vi "Calculate Legend String Origin Point.vi"(8 "error in (no error)":errorcluster caption="错误输入（无错误）", 9 "origin":cluster{"x":i16, "y":i16} caption="Origin", 10 "Legend Info":T1={"Name"="", "Percent"=0.0, "TxtColor"=0, "Hor Space"=0, "Ver Space"=5, "Color Segement"=[16448250, 0, 16736786, 1198079]}, 11 "Gradient PieChart 输入":refnum<class "Gradient PieChart.lvclass"> caption="DNL_LabVIEW Object in") -> (0 "error out":errorcluster caption="错误输出", 1 "Next Origin":cluster{"x":i16, "y":i16} caption="Next Orgin", 3 "Gradient PieChart 输出":refnum<class "Gradient PieChart.lvclass"> caption="DNL_LabVIEW Object out")   [LabVIEW 2012, in "Picture Box Tools.lvlib" / "Gradient PieChart.lvclass"]
uses:
  Gradient PieChart.lvclass
  Legend Info.ctl
  Picture Box Tools.lvlib
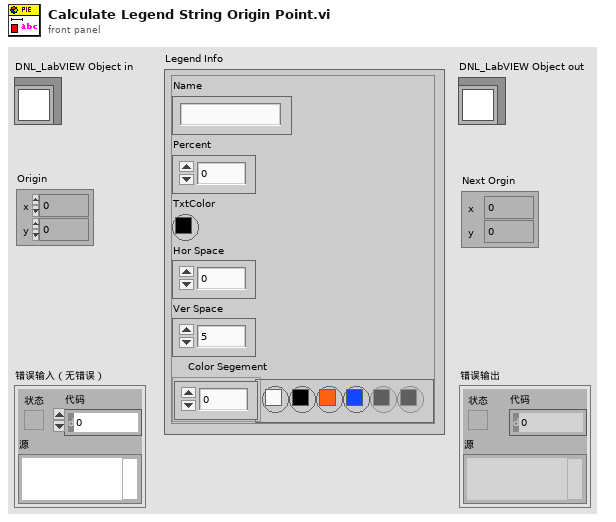
[diagram p1: front panel]
types:
  T1 = typedef "Picture Box Tools.lvlib/Gradient PieChart.lvclass/Legend Info.ctl" = cluster{"Name":string, "Percent":dbl, "TxtColor":u32, "Hor Space":i16, "Ver Space":i16, "Color Segement":u32[]}
  T2 = cluster{"left":i16, "top":i16, "right":i16, "bottom":i16}
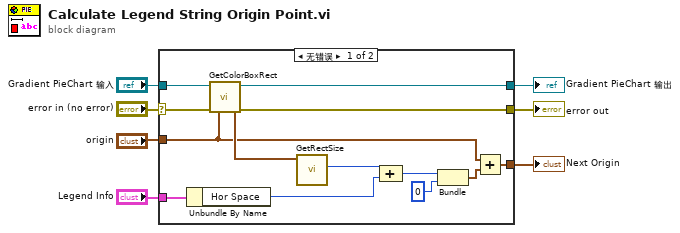
[diagram p0: block diagram]
diagram:
  n1 = case shown="无错误" "error in (no error)" {
    selector: "error in (no error)" -> [w17 w22]
    tunnel: [w16 w22] -> w6
    tunnel: [w18 w21] -> w4
    tunnel: "Gradient PieChart 输入" -> [w19 w21]
    tunnel: "Legend Info" -> [w20 _]
    tunnel: "origin" -> [w11 _]
    tunnel: [w10 _] -> w1
    frame No Error {
      n2 = Unbundle By Name(w20) -> ("Hor Space"=w14:i16)
      n3 = call "GetColorBoxRect.vi"("error in (no error)"=w17, "origin"=w11, "Gradient PieChart 输入"=w19) -> ("error out"=w16:errorcluster, "ColorBoxRect"=w15:T2, "Gradient PieChart 输出"=w18:refnum<class "Gradient PieChart.lvclass">)  [unwired: 6 in]
      n4 = call "GetRectSize.vi"("rect"=w15) -> ("Width"=w8:i16)  [unwired: 7 in, 3 out]
      n5 = Compound Arithmetic op=ADD(w8, w14) -> (w13:i16)
      n6 = Bundle(w13, i16 0) -> (w12:cluster{i16, i16})  [unwired: 1 in]
      n7 = Add(x=w11, y=w12) -> (x+y=w10:cluster{i16, i16})
    }
    frame Error {
    }
  }
  "error out" <- w6
  "Gradient PieChart 输出" <- w4
  "Next Origin" <- w1
